vi "Instrument.KH7008.TestLauncher.vi"() -> ()   [LabVIEW 2019, in "Instrument.KH7008.lvclass"]
uses:
  Instrument.KH7008.lvclass
  <vilib>/JKI/JKI SMO/SMO/Typedefs/SMOState --Enum.ctl
  C:/Program Files (x86)/National Instruments/LabVIEW 2019/vi.lib/JKI/JKI SMO/SMO/SMO.lvclass
  <vilib>/JKI/JKI SMO/SMO/SMO.lvclass
panel:
  out "SMO State":T1
  out "error out":errorcluster
  in  "Stop":bool
  # "Basic SMO Test Launcher"
  # "For instructions on how to use the JKI State Machine Objects, examples and video tutorials, visit:\nhttp://jki.net/state-machine-objects/\n\nJKI State Machine Objects™\nhttp://jki.net/state-machine-objects/\nCopyright (C) 2005-2015, JKI <info@jki.net>\nALL RIGHTS RESERVED"
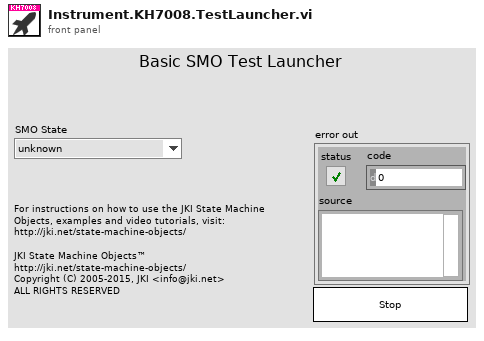
[diagram p1: front panel]
types:
  T1 = typedef "SMO.lvclass/SMOState --Enum.ctl" = enum16{"unknown", "Created", "Started", "Stopped"}
  T2 = typedef "SMO.lvclass/Public Events.ctl" = cluster{"Error":refnum<user-event>, "State":refnum<user-event>, "Reserve State":refnum<user-event>}
  T3 = cluster{"Event Registration Refnum":refnum<event-registration>}
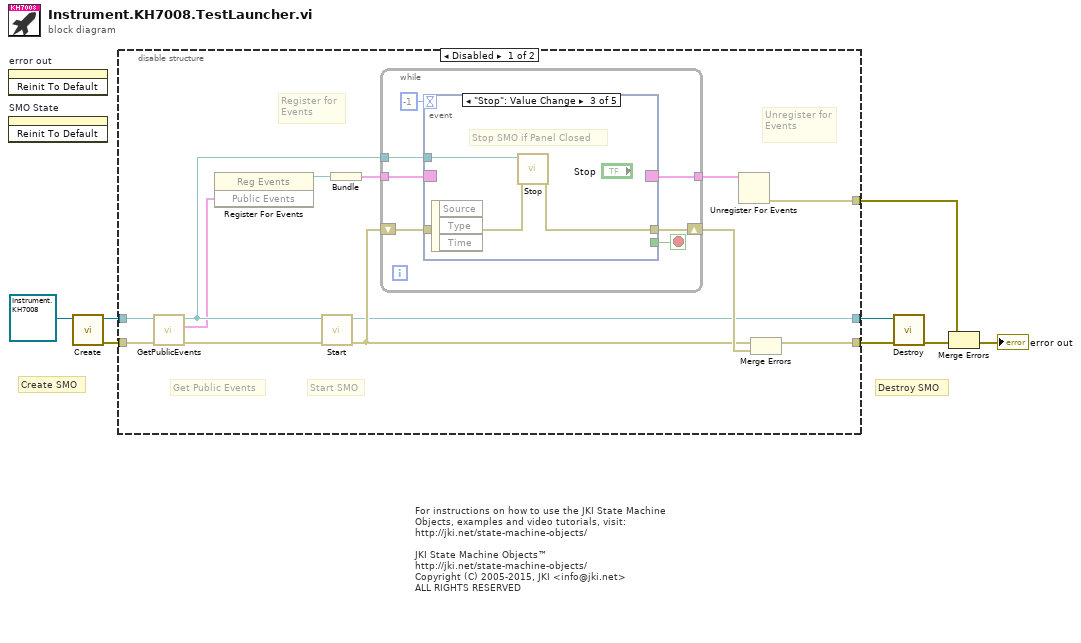
[diagram p0: block diagram]
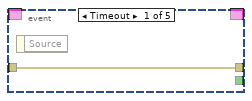
[diagram p2: hidden frame]
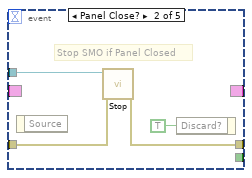
[diagram p3: hidden frame]
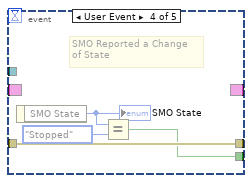
[diagram p4: hidden frame]
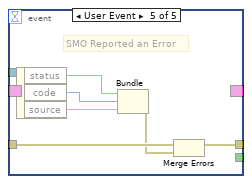
[diagram p5: hidden frame]
diagram:
  # "For instructions on how to use the JKI State Machine Objects, examples and video tutorials, visit:\nhttp://jki.net/state-machine-objects/\n\nJKI State Machine Objects™\nhttp://jki.net/state-machine-objects/\nCopyright (C) 2005-2015, JKI <info@jki.net>\nALL RIGHTS RESERVED"
  # "Destroy SMO"
  # "Create SMO"
  n1 = invoke on="error out" class="Clust (strict)" method="Reinit To Default"() -> ()  [unwired: 3 in, 3 out]
  n2 = invoke on="SMO State" class="Enum (strict)" method="Reinit To Default"() -> ()  [unwired: 3 in, 3 out]
  n3 = call <vilib>:"Create.vi"("SMO"=refnum<class "Instrument.KH7008.lvclass"> refnum ("SMO.Template.lvclass")) -> ("error out"=w1:errorcluster, "SMO out"=w2:refnum<class "Instrument.KH7008.lvclass">)  [unwired: 8 in, 1 out]
  n4 = disable-structure shown="Disabled" {
    disable-tunnel: [w18 _] -> w8
    disable-tunnel: [w16 _] -> w4
    disable-tunnel: [w15 _] -> w3
    disable-tunnel: w2 -> [w14 _]
    disable-tunnel: w1 -> [w13 _]
    frame Disabled {
      # "Get Public Events"
      # "Start SMO"
      # "Unregister for Events"
      # "Register for Events"
      n5 = call <vilib>:"GetPublicEvents.vi"("error in (no error)"=w13, "SMO"=w14) -> ("error out"=w12:errorcluster, "Public Events"=w10:T2, "SMO out"=w11:refnum<class "Instrument.KH7008.lvclass">)  [unwired: 7 in]
      n6 = register-events(w10) -> (reference out=w9:refnum<event-registration>)  [unwired: 2 in, 1 out]
      n7 = call <vilib>:"Start.vi"("error in (no error)"=w12, "SMO"=w11) -> ("error out"=w17:errorcluster, "SMO out"=w15:refnum<class "Instrument.KH7008.lvclass">)  [unwired: 8 in]
      n8 = Bundle("Event Registration Refnum"=w9) -> (w20:T3)  [unwired: 1 in]
      n9 = while {
        shift-right: [w27] -> w19
        shift-left: w17 -> [w26]
        tunnel: w20 -> [w25]
        tunnel: [w24] -> w21
        tunnel: w11 -> [w23]
        stop <- w28 stop-if-true
        n10 = event shown="[2] \"Stop\": Value Change" {
          selector: w25 -> [_ _ _ _ _]
          dyn-events: [_ _ _ _ _] -> w24
          timeout: -1 -> [_ _ _ _ _]
          tunnel: [_ _ _ w37 _] -> w28
          tunnel: w23 -> [_ w33 w36 _ _]
          tunnel: [w29 w32 w35 w40 w44] -> w27
          tunnel: w26 -> [w29 w31 w34 w40 w42]
          event Timeout {
            n11 = event-data() -> ()  [unwired: 1 in, 1 out]
          }
          event Panel Close? {
            # "Stop SMO if Panel Closed"
            n12 = event-data() -> ()  [unwired: 1 in, 1 out]
            n13 = call <vilib>:"Stop.vi"("error in (no error)"=w31, "SMO"=w33) -> ("error out"=w32:errorcluster)  [unwired: 8 in, 1 out]
            n14 = event-data("Discard?"=TRUE ("OK")) -> ()  [unwired: 1 in, 1 out]
          }
          event "Stop": Value Change {
            # "Stop SMO if Panel Closed"
            n15 = event-data() -> ()  [unwired: 1 in, 3 out]
            n16 = call <vilib>:"Stop.vi"("error in (no error)"=w34, "SMO"=w36) -> ("error out"=w35:errorcluster)  [unwired: 8 in, 1 out]
          }
          event User Event {
            # "SMO Reported a Change\nof State"
            n17 = event-data() -> ("SMO State"=w39:T1)  [unwired: 1 in]
            "SMO State" <- w39
            n18 = Equal?(x=w39, y=SMOState_--Enum."Stopped") -> (x = y?=w37:bool)
          }
          event User Event {
            # "SMO Reported an Error"
            n19 = event-data() -> ("status"=w43:bool, "code"=w46:i32, "source"=w45:string)  [unwired: 1 in]
            n20 = Bundle("status"=w43, "code"=w46, "source"=w45) -> (w41:errorcluster)  [unwired: 1 in]
            n21 = Merge Errors(w42, w41) -> (w44:errorcluster)
          }
        }
      }
      n22 = Unregister For Events(event registration refnum=w21) -> (error out=w18:errorcluster)  [unwired: 1 in]
      n23 = Merge Errors(w17, w19) -> (w16:errorcluster)
    }
    frame Enabled {
    }
  }
  n24 = call <vilib>:"Destroy.vi"("error in (no error)"=w4, "SMO"=w3) -> ("error out"=w6:errorcluster)  [unwired: 9 in]
  n25 = Merge Errors(w8, w6) -> (→"error out":errorcluster)
